vi "CommandHistory.vi"(10 "CommandVI":string, 11 "QueueIn":refnum<queue>) -> (2 "SecondsSince1Jan1904":timestamp, 3 "HiStory":string[](array[string]))   [LabVIEW 2021, in "YActor.lvclass"]
uses:
  YActor.lvclass
  YActor.lvclass/YActor.ctl
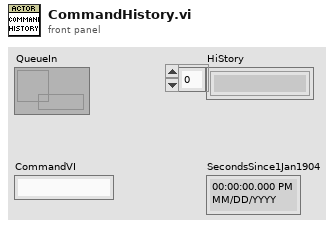
[diagram p1: front panel]
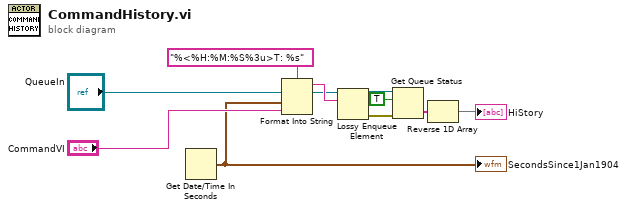
[diagram p0: block diagram]
diagram:
  n1 = Get Date/Time In Seconds() -> (seconds since 1Jan1904=w1:timestamp)
  "SecondsSince1Jan1904" <- w1
  n2 = Format Into String(format string="%<%H:%M:%S%3u>T: %s", w1, "CommandVI") -> (resulting string=w7:string)  [unwired: 2 in, 1 out]
  n3 = Lossy Enqueue Element(queue="QueueIn", element=w7) -> (queue out=w3:refnum<queue>, error out=w10:errorcluster)  [unwired: 1 in, 2 out]
  n4 = Get Queue Status(queue=w3, return elements? (F)=TRUE, error in (no error)=w10) -> (elements=w5:string[])  [unwired: 7 out]
  n5 = Reverse 1D Array(array=w5) -> (reversed array=→"HiStory":string[])
